vi "Secondary Driver.vi"(7 "Primary Driver":T2, 10 "Robot Global Data In":T1, 11 "Secondary Driver":T2) -> (3 "Robot Global Data Out":T1)   [LabVIEW 2013]
uses:
  Team Code/Robot Global Data.vi
  <vilib>/Rock Robotics/WPI/Solenoid/WPI_SolenoidValue.ctl
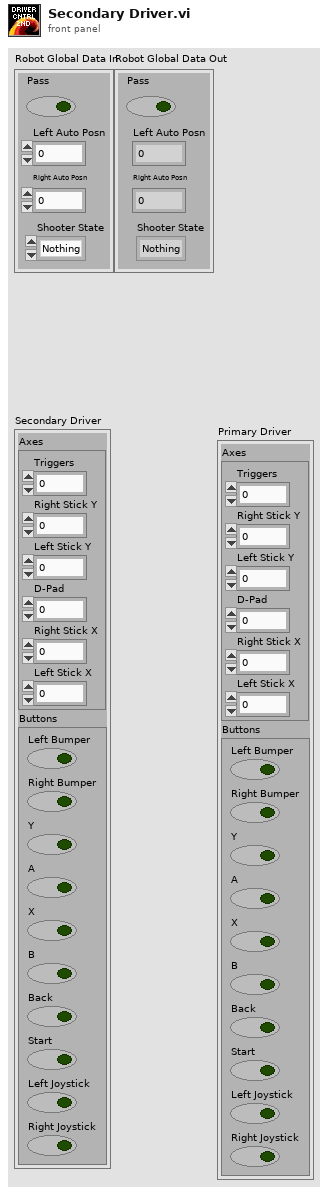
[diagram p1: front panel]
types:
  T1 = cluster{"Left Auto Posn":dbl, "Right Auto Posn":dbl, "Pass":bool, "Shooter State":enum16{"Nothing", "Fire", "Load"}}
  T2 = cluster{"Axes":cluster{"Triggers":dbl, "Right Stick Y":dbl, "Left Stick Y":dbl, "D-Pad":dbl, "Right Stick X":dbl, "Left Stick X":dbl}, "Buttons":cluster{"Left Bumper":bool, "Right Bumper":bool, "Y":bool, "A":bool, "X":bool, "B":bool, "Back":bool, "Start":bool, "Left Joystick":bool, "Right Joystick":bool}}
  T3 = typedef "WPI_SolenoidValue.ctl" = enum16{"Off", "On", "Forward", "Reverse"}
  T4 = enum16{"Loader Up", "Loader Down", "Ball In Possesion"}
  T5 = cluster{"Left Power":dbl, "Right Power":dbl, "Shooter State":enum16{"Nothing", "Fire", "Load"}, "Loader State":enum16{"Loader Up", "Loader Down", "Ball In Possesion"}, "Auto Time":dbl, "Tele Time":dbl, "Driver":dbl, "Not Allowed":bool, "Right Speed":dbl, "Left Speed":dbl}
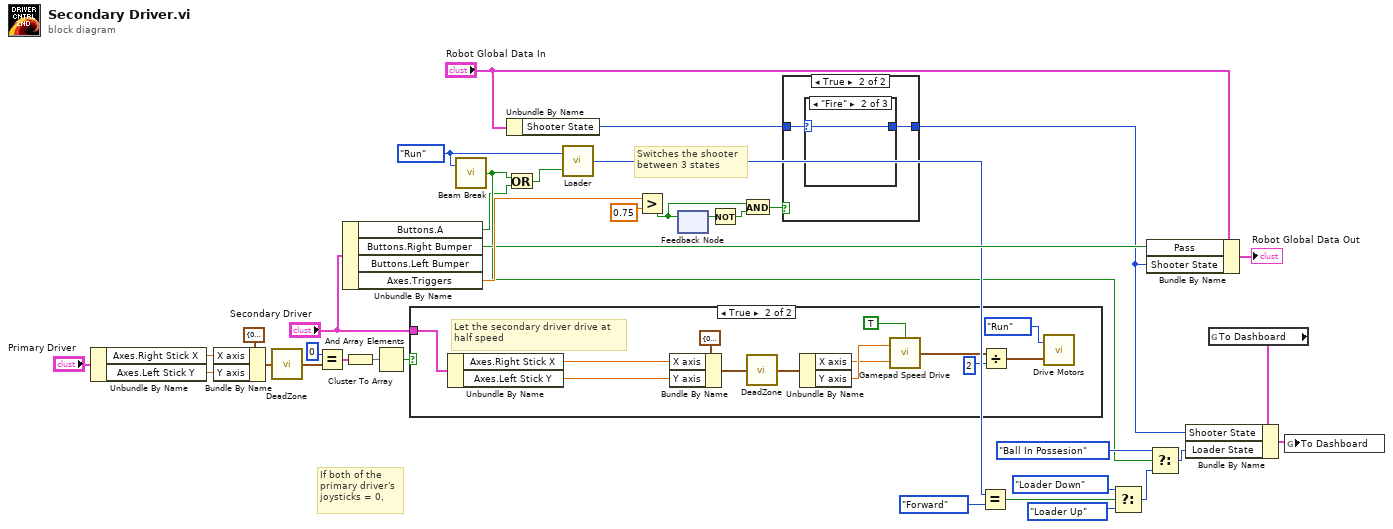
[diagram p0: block diagram]
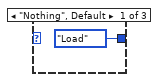
[diagram p3: hidden frame]
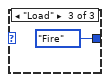
[diagram p4: hidden frame]
diagram:
  w15 = enum16{"Start", "Run", "End"}."Run" ("Enum")
  # "Switches the shooter\nbetween 3 states"
  # "If both of the\nprimary driver's\njoysticks = 0,"
  n1 = Unbundle By Name("Primary Driver") -> ("Axes.Right Stick X"=w36:dbl, "Axes.Left Stick Y"=w35:dbl)
  n2 = Bundle By Name(cluster=cluster{"X axis":dbl, "Y axis":dbl} {"X axis"=0.0, "Y axis"=0.0} ("Drive Axes"), "X axis"=w36, "Y axis"=w35) -> (w34:cluster{"X axis":dbl, "Y axis":dbl})
  n3 = call "DeadZone.vi"("Drive Axes"=w34) -> ("Drive Axes"=w31:cluster{"X axis":dbl, "Y axis":dbl})
  n4 = Equal?(x=0, y=w31) -> (x = y?=w30:cluster{"X axis":bool, "Y axis":bool})
  n5 = Unbundle By Name("Secondary Driver") -> ("Buttons.A"=w1:bool, "Buttons.Right Bumper"=w23:bool, "Axes.Triggers"=w25:dbl)  [unwired: 1 out]
  n6 = Cluster To Array(cluster=w30) -> (array=w28:bool[])
  n7 = And Array Elements(Boolean array=w28) -> (logical AND=w27:bool)
  n8 = case shown="True" w27 {
    tunnel: "Secondary Driver" -> [_ w44]
    frame False {
    }
    frame True {
      # "Let the secondary driver drive at \nhalf speed"
      n9 = Unbundle By Name(w44) -> ("Axes.Right Stick X"=w47:dbl, "Axes.Left Stick Y"=w46:dbl)
      n10 = Bundle By Name(cluster=cluster{"X axis":dbl, "Y axis":dbl} {"X axis"=0.0, "Y axis"=0.0} ("Drive Axes"), "X axis"=w47, "Y axis"=w46) -> (w45:cluster{"X axis":dbl, "Y axis":dbl})
      n11 = call "DeadZone.vi"("Drive Axes"=w45) -> ("Drive Axes"=w40:cluster{"X axis":dbl, "Y axis":dbl})
      n12 = Unbundle By Name(w40) -> ("X axis"=w38:dbl, "Y axis"=w39:dbl)
      n13 = call "Gamepad Speed Drive.vi"("Quick Turn"=TRUE, "Turn"=w38, "Speed"=w39) -> ("Motor Powers"=w41:cluster{"RMotor":dbl, "LMotor":dbl})
      n14 = Divide(x=w41, y=2) -> (x/y=w42:cluster{"RMotor":dbl, "LMotor":dbl})
      n15 = call "Drive Motors.vi"("Motor Powers"=w42, "Enum"=enum16{"Start", "Run", "End"}."Run") -> ()
    }
  }
  n16 = call "Beam Break.vi"("Enum"=w15) -> ("Broken"=w3:bool)  [unwired: 1 in]
  n17 = Unbundle By Name("Robot Global Data In") -> ("Shooter State"=w20:enum16{"Nothing", "Fire", "Load"})
  n18 = Or(x=w3, y=w1) -> (x .or. y?=w2:bool)
  n19 = call "Loader.vi"("Down (Forward)"=w2, "Enum"=w15) -> ("State"=w8:T3)
  n20 = Greater?(x=w25, y=0.75) -> (0:w16:bool)
  n21 = feedback-in #1(w16) -> ()
  n22 = feedback #1() -> (w17:bool)  [unwired: 1 in]
  n23 = Not(x=w17) -> (.not. x?=w18:bool)
  n24 = And(x=w16, y=w18) -> (x .and. y?=w19:bool)
  n25 = case shown="True" w19 {
    tunnel: w20 -> [w50 w52]
    tunnel: [w50 w51] -> w13
    frame False {
    }
    frame True {
      n26 = case shown="\"Fire\"" w52 {
        selector: w52 -> [_ w54 _]
        tunnel: [enum16{"Nothing", "Fire", "Load"}."Load" ("Shooter State") w54 enum16{"Nothing", "Fire", "Load"}."Fire" ("Shooter State")] -> w51
        frame "Nothing", Default {
        }
        frame "Fire" {
        }
        frame "Load" {
        }
      }
    }
  }
  n27 = Equal?(x=w8, y=WPI_SolenoidValue."Forward") -> (x = y?=w6:bool)
  n28 = Select(t=T4."Loader Down" ("Loader State"), s=w6, f=T4."Loader Up" ("Loader State")) -> (s? t:f=w11:T4)
  n29 = Bundle By Name(cluster="Robot Global Data In", "Pass"=w23, "Shooter State"=w13) -> (→"Robot Global Data Out":T1)
  n30 = Select(t=T4."Ball In Possesion" ("Loader State"), s=w3, f=w11) -> (s? t:f=w5:T4)
  n31 = global read "Robot Global Data.vi" "To Dashboard"() -> (w14:T5)
  n32 = Bundle By Name(cluster=w14, "Shooter State"=w13, "Loader State"=w5) -> (w4:T5)
  n33 = global write "Robot Global Data.vi" "To Dashboard"(w4) -> ()
